vi "interfazlabviewcarrito.vi"() -> ()   [LabVIEW 2023]
uses:
  <vilib>/Instr/_visa.llb/VISA Configure Serial Port (Instr).vi
  <vilib>/Utility/file.llb/Write Delimited Spreadsheet (DBL).vi
  <vilib>/regexp/Match Regular Expression.xnode
panel:
  out "Waveform Chart 2":dbl[][](graph)
  out "x2":dbl
  out "x1":dbl
  out "Referencia":dbl
  out "Distancia":dbl
  out "Datos a tomar del serial":string
  out "Datos seriales del arduino":string
  out "Waveform Chart":dbl[][](graph)
  out "error out":errorcluster
  in  "stop":bool
  in  "REFERENCIA":dbl
  in  "VISA resource name":refnum<visa-resource-name>
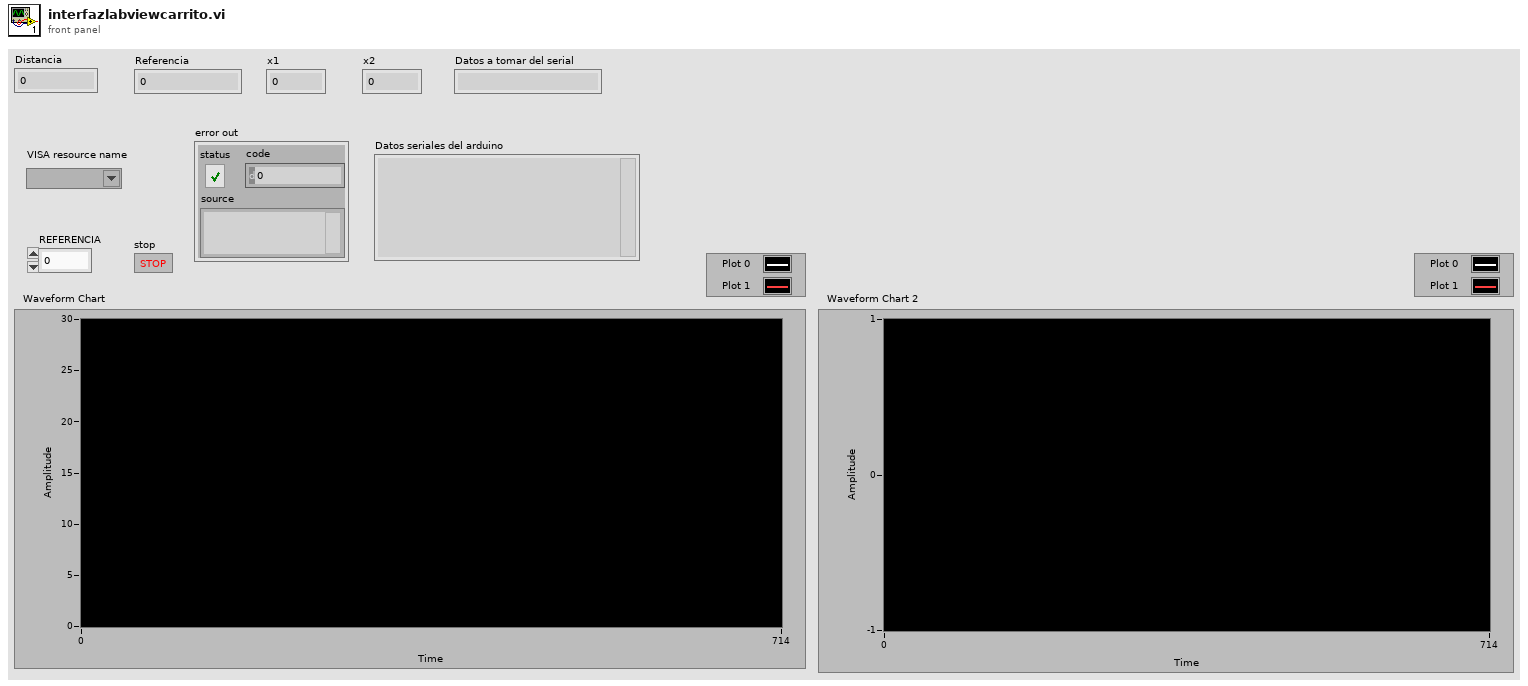
[diagram p1: front panel]
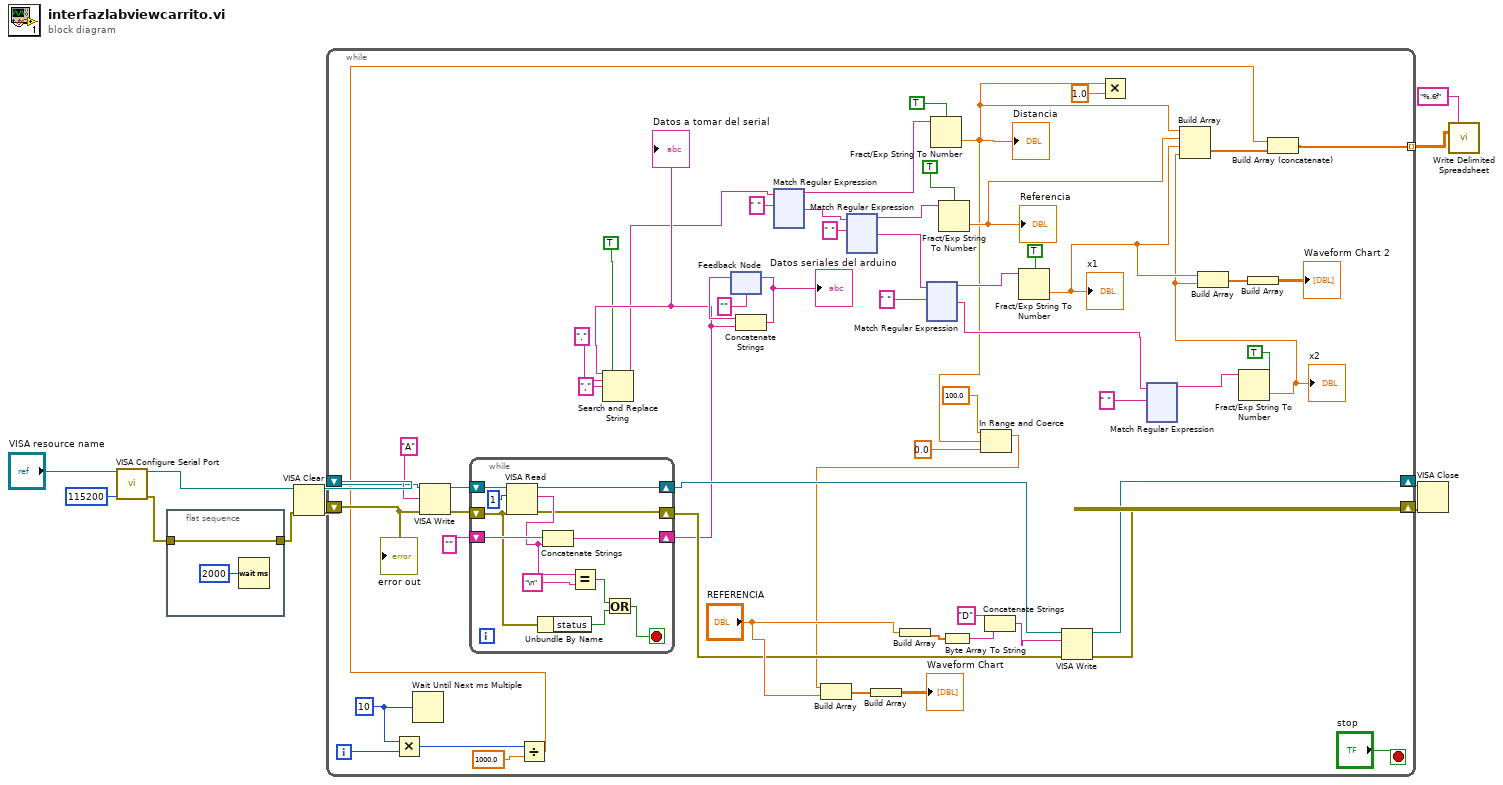
[diagram p0: block diagram]
diagram:
  n1 = call-poly "VISA Configure Serial Port"("VISA resource name"="VISA resource name", "baud rate (9600)"=u32 115200) -> ("VISA resource name out"=w7:refnum<visa-resource-name>, "error out"=w10:errorcluster)  [unwired: 12 in]
  n2 = flat-sequence {
    tunnel: w10 -> [w12]
    tunnel: [w12] -> w5
    frame #0 {
      n3 = Wait (ms)(milliseconds to wait=u32 2000) -> ()  [unwired: 1 out]
    }
  }
  n4 = VISA Clear(VISA resource name=w7, error in (no error)=w5) -> (VISA resource name out=w6:refnum<visa-resource-name>, error out=w4:errorcluster)
  n5 = while {
    shift-right: [w66] -> w9
    shift-left: w6 -> [w61]
    shift-right: [w65] -> w8
    shift-left: w4 -> [w60]
    tunnel: [w21] -> w2 mode=indexing
    i -> [w22]
    stop <- "stop" stop-if-true
    w25 = u32 10 ("millisecond multiple")
    n6 = Multiply(x=w25, y=w22) -> (x*y=w23:u32)
    n7 = Wait Until Next ms Multiple(millisecond multiple=w25) -> ()  [unwired: 1 out]
    n8 = VISA Write(VISA resource name=w61, write buffer="A", error in (no error)=w60) -> (VISA resource name out=w54:refnum<visa-resource-name>, error out=w53:errorcluster)  [unwired: 1 out]
    n9 = while {
      shift-right: [w541] -> w51
      shift-left: w54 -> [w551]
      shift-right: [w540] -> w52
      shift-left: w53 -> [w545]
      shift-right: [w549] -> w46
      shift-left: "" -> [w548]
      stop <- w542 stop-if-true
      n10 = VISA Read(VISA resource name=w551, byte count=u32 1, error in (no error)=w545) -> (VISA resource name out=w541:refnum<visa-resource-name>, read buffer=w547:string, error out=w540:errorcluster)  [unwired: 1 out]
      n11 = Unbundle By Name(w545) -> ("status"=w543:bool)
      n12 = Concatenate Strings(w548, w547) -> (w549:string)
      n13 = Equal?(x=w547, y="\n") -> (x = y?=w544:bool)
      n14 = Or(x=w544, y=w543) -> (x .or. y?=w542:bool)
    }
    "Datos a tomar del serial" <- w46
    n15 = Divide(x=w23, y=1000.0) -> (x/y=w19:dbl)
    n16 = Search and Replace String(replace all?=TRUE ("replace all? (F)"), input string=w46, search string="." ("substring (\"\")"), replace string="," ("replace string (\"\")")) -> (result string=w42:string)  [unwired: 4 in, 3 out]
    n17 = feedback #1("") -> (w57:string)
    n18 = Concatenate Strings(w57, w46) -> (w58:string)
    "Datos seriales del arduino" <- w58
    n19 = feedback-in #1(w58) -> ()
    n20 = xnode "Match Regular Expression"("input string"=w42, "regular expression"=" ") -> ("before match"=w41:string, "after match"=w48:string)  [unwired: 4 in, 3 out]
    n21 = xnode "Match Regular Expression"("input string"=w48, "regular expression"=" ") -> ("before match"=w39:string, "after match"=w36:string)  [unwired: 4 in, 3 out]
    n22 = Build Array("REFERENCIA") -> (w70:dbl[])
    n23 = xnode "Match Regular Expression"("input string"=w36, "regular expression"=" ") -> ("before match"=w38:string, "after match"=w31:string)  [unwired: 4 in, 3 out]
    n24 = Fract/Exp String To Number(use system decimal point (T)=TRUE, string=w41) -> (number=w18:dbl)  [unwired: 2 in, 1 out]
    "Distancia" <- w18
    n25 = Fract/Exp String To Number(use system decimal point (T)=TRUE, string=w39) -> (number=w30:dbl)  [unwired: 2 in, 1 out]
    "Referencia" <- w30
    n26 = Byte Array To String(unsigned byte array=w70) -> (string=w69:string)
    n27 = In Range and Coerce(upper limit=100.0, x=w18, lower limit=0.0) -> (coerced(x)=w26:dbl)  [unwired: 1 out]
    n28 = Build Array(w26, "REFERENCIA") -> (w62:dbl[])
    n29 = Build Array(w62) -> (→"Waveform Chart":dbl[][])
    n30 = Concatenate Strings("D" ("string"), w69) -> (w67:string)
    n31 = Fract/Exp String To Number(use system decimal point (T)=TRUE, string=w38) -> (number=w15:dbl)  [unwired: 2 in, 1 out]
    "x1" <- w15
    n32 = VISA Write(VISA resource name=w51, write buffer=w67, error in (no error)=w52) -> (VISA resource name out=w66:refnum<visa-resource-name>, error out=w65:errorcluster)  [unwired: 1 out]
    n33 = Multiply(x=w18, y=1.0) -> ()  [unwired: 1 out]
    n34 = xnode "Match Regular Expression"("input string"=w31, "regular expression"=" ") -> ("before match"=w34:string)  [unwired: 4 in, 4 out]
    n35 = Fract/Exp String To Number(use system decimal point (T)=TRUE, string=w34) -> (number=w14:dbl)  [unwired: 2 in, 1 out]
    "x2" <- w14
    n36 = Build Array(w18, w30, w15, w14) -> (w20:dbl[])
    n37 = Build Array(w15, w14) -> (w16:dbl[])
    n38 = Build Array(w16) -> (→"Waveform Chart 2":dbl[][])
    n39 = Build Array (concatenate)(w19, w20) -> (w21:dbl[])
    "error out" <- w60
  }
  n40 = VISA Close(VISA resource name=w9, error in (no error)=w8) -> ()  [unwired: 1 out]
  n41 = call-poly <vilib>:"Write Delimited Spreadsheet.vi"("format (%.3f)"="%.6f", "2D data"=w2) -> ()  [unwired: 12 in, 2 out]
